vi "DrivePath-C.vi"(11 "Params":string[][](array[string])) -> ()   [LabVIEW 2019]
uses:
  Dawgma Programming Library/Controls/PurePursuit/PathFileData.ctl
  Dawgma Programming Library/Controls/PurePursuit/RobotNeededPathData.ctl
  Framework/Robot Global Data.vi
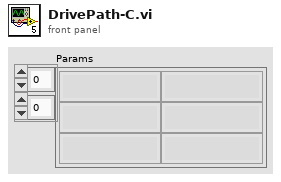
[diagram p1: front panel]
types:
  T1 = typedef "PathFileData.ctl" = cluster{"RobotNeeded":T2, "Meta":cluster{"Path (px)":cluster{i32, i32}[], "RobotWidth":dbl, "RobotLength":dbl, "CenterOfRotYOffset":dbl, "Roundedness":dbl, "StartingPositionPreset":u32}}
  T2 = typedef "RobotNeededPathData.ctl" = cluster{"Path":cluster{dbl, dbl}[], "MaxVel":dbl, "MaxAccel":dbl, "Backwards?":bool, "PointSpacing":dbl, "LookaheadDist":dbl, "Speed/Curve":dbl, "SlowDistanceAtEnd":dbl, "SlowSpeed":dbl, "MaxDeAccel":dbl}
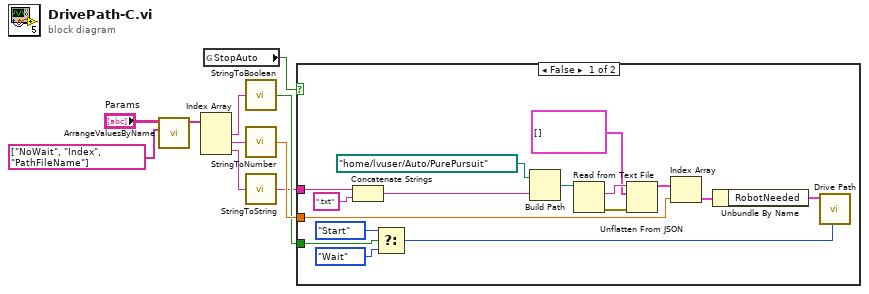
[diagram p0: block diagram]
diagram:
  n1 = call "ArrangeValuesByName.vi"("Names"=string[] ["NoWait", "Index", "PathFileName"], "Names/Values in"="Params") -> ("Values Out"=w4:string[])  [unwired: 9 in]
  n2 = Index Array(array=w4) -> (element #1=w3:string, element #2=w2:string, element #3=w1:string)  [unwired: 3 in]
  n3 = global read "Robot Global Data.vi" "StopAuto"() -> (w10:bool)
  n4 = call "StringToBoolean.vi"("String"=w3) -> ("Output"=w8:bool)
  n5 = call "StringToNumber.vi"("String"=w2) -> ("Output"=w9:dbl)
  n6 = call "StringToString.vi"("String"=w1) -> ("Output"=w7:string)
  n7 = case shown="False" w10 {
    tunnel: w9 -> [w17 _]
    tunnel: w8 -> [w11 _]
    tunnel: w7 -> [w26 _]
    frame False {
      n8 = Concatenate Strings(w26, ".txt" ("string")) -> (w24:string)
      n9 = Select(t=enum16{"Start", "Wait"}."Start" ("Synchronization"), s=w11, f=enum16{"Start", "Wait"}."Wait" ("Synchronization")) -> (s? t:f=w12:enum16{"Start", "Wait"})
      n10 = Build Path(base path=path "/home/lvuser/Auto/PurePursuit", name or relative path=w24) -> (appended path=w22:path)
      n11 = Read from Text File(file (use dialog)=w22) -> (text=w20:string, error out=w21:errorcluster)  [unwired: 3 in, 2 out]
      n12 = Unflatten From JSON(JSON string=w20, type and defaults=T1[] [], error in (no error)=w21) -> (value=w18:T1[])  [unwired: 4 in, 1 out]
      n13 = Index Array(array=w18, index=w17) -> (element=w16:T1)
      n14 = Unbundle By Name(w16) -> ("RobotNeeded"=w15:T2)
      n15 = call "Drive Path.vi"("Synchronication"=w12, "RobotNeededPathData"=w15) -> ()  [unwired: 9 in, 1 out]
    }
    frame True {
    }
  }
